vi "WSVCAP SHL Host TL I2C Read.vi"(0 "Bytes to Read":u8=8, 5 "Sub Address [U8]":u8=191 format="%.0x", 7 "Socket Mask [U64]":u64 format="%016x", 11 "error in":errorcluster, 13 "Log (T)":bool=TRUE, 14 "FPGA":T1) -> (4 "C Read Data Out":u8[][](array[numeric]) format="%.0x", 15 "error out":errorcluster)   [LabVIEW 2017]
uses:
  Type Defs/WSVCAP SHL FPGA Enum.ctl
  Type Defs/WSVCAP SHL Function Enum.ctl
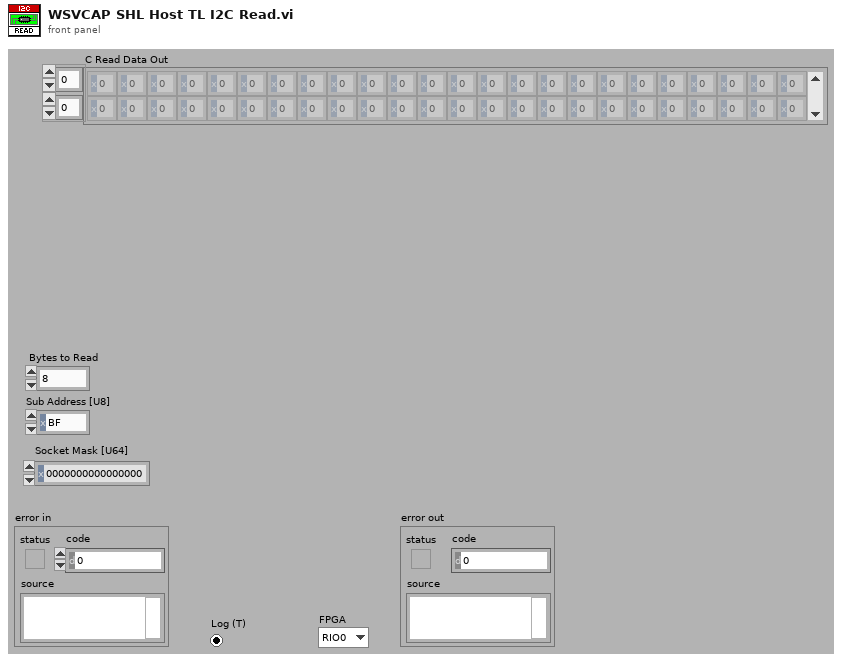
[diagram p1: front panel]
types:
  T1 = typedef "WSVCAP SHL FPGA Enum.ctl" = enum16{"RIO0", "RIO1"}
  T2 = typedef "WSVCAP SHL Function Enum.ctl" = enum16{"Initialize", "Configure I2C", "Configure RFFE", "Write I2C", "Read I2C", "Write RFFE", "Read RFFE", "Start RFFE Cycle", "Stop RFFE Cycle", "Get Status", "Close"}
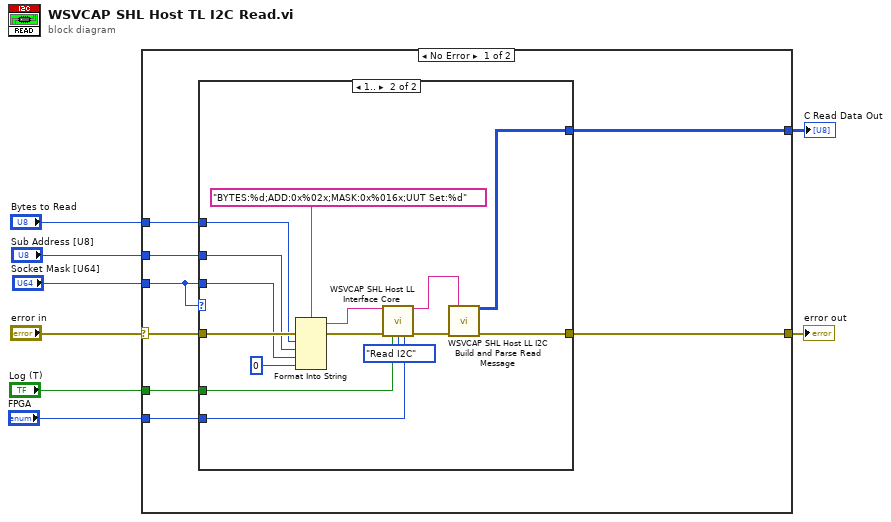
[diagram p0: block diagram]
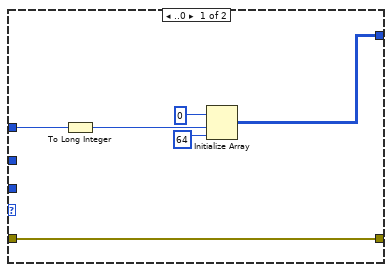
[diagram p2: hidden frame]
diagram:
  n1 = case shown="No Error" "error in" {
    selector: "error in" -> [w15 w38]
    tunnel: [w16 w38] -> w7
    tunnel: [w9 _] -> w2
    tunnel: "Bytes to Read" -> [w14 _]
    tunnel: "Sub Address [U8]" -> [w13 _]
    tunnel: "Socket Mask [U64]" -> [w12 _]
    tunnel: "Log (T)" -> [w11 _]
    tunnel: "FPGA" -> [w10 _]
    frame No Error {
      n2 = case shown="1.." w12 {
        tunnel: [w22 w36] -> w16
        tunnel: [w17 w34] -> w9
        tunnel: w15 -> [w22 w33]
        tunnel: w14 -> [w19 w30]
        tunnel: w13 -> [_ w29]
        tunnel: w12 -> [_ w28]
        tunnel: w11 -> [_ w25]
        tunnel: w10 -> [_ w24]
        frame ..0 {
          n3 = To Long Integer(number=w19) -> (32bit integer=w18:i32)
          n4 = Initialize Array(u8 0 ("Read Data"), w18, 64 ("Read Data")) -> (w17:u8[][])
        }
        frame 1.. {
          n5 = Format Into String(format string="BYTES:%d;ADD:0x%02x;MASK:0x%016x;UUT Set:%d", error in=w33, w30, w29, w28, 0 ("input 4")) -> (resulting string=w27:string, error out=w32:errorcluster)  [unwired: 1 in]
          n6 = call "WSVCAP SHL Host LL Interface Core.vi"("Message In"=w27, "error in"=w32, "Log (T)"=w25, "Function"=WSVCAP_SHL_Function_Enum."Read I2C", "FPGA"=w24) -> ("Message Out"=w35:string, "error out"=w37:errorcluster)  [unwired: 8 in, 1 out]
          n7 = call "WSVCAP SHL Host LL I2C Build and Parse Read Message.vi"("Message In"=w35, "error in"=w37) -> ("C1 Read Data Out"=w34:u8[][], "error out"=w36:errorcluster)  [unwired: 10 in, 2 out]
        }
      }
    }
    frame Error {
    }
  }
  "error out" <- w7
  "C Read Data Out" <- w2
